vi "2025_day1.vi"() -> ()   [LabVIEW 2025]
uses:
  <userlib>/_OpenG.lib/string/string.llb/openg_string.lvlib
panel:
  out "Task 2":i32
  out "Task 1":i32
  in  "Switch":bool caption="Ex. Data  vs.  User Data"
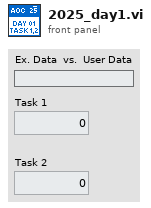
[diagram p1: front panel]
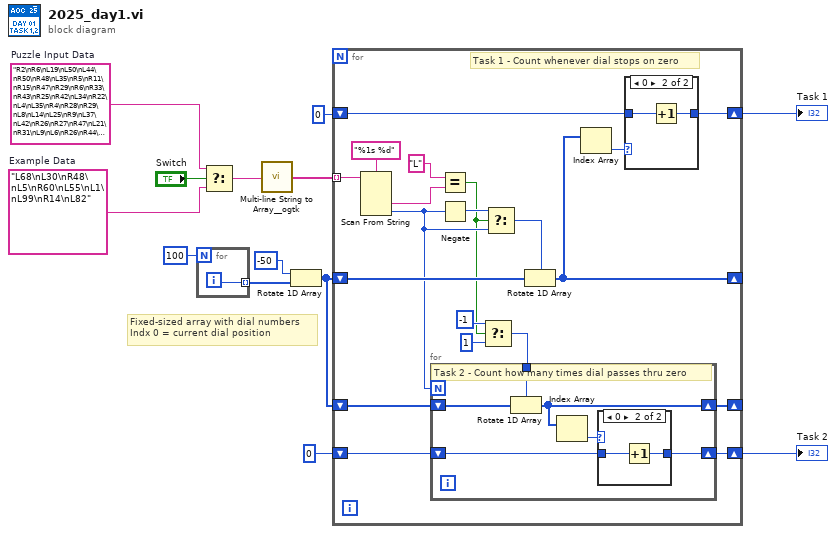
[diagram p0: block diagram]
diagram:
  w11 = "R2\nR6\nL19\nL50\nL44\nR50\nR48\nL35\nR5\nR11\nR15\nR47\nR29\nR6\nR33\nR43\nR25\nR42\nL34\nR22\nL4\nL35\nR4\nR28\nR29\nL8\nL14\nL25\nR9\nL37\nL42\nR26\nR27\nR47\nL21\nR31\nL9\nL6\nR26\nR44\nR2\nL38\nL14\nR21\nR49\nL47\nR23\nL25\nR20\nL13\nR12\nL46\nL66\nR12\nL41\nL92\nR19\nL89\nR30\nL39\nL30\nL24\nR13\nR75\nL92\nR58\nR68\nR32\nR12\nL33\nR49\nL28\nR41\nR24\nR76\nL62\nR14\nL93\nR25\nR75\nR68\nL19\nL49\nR13\nR71\nR16\nL4\nL40\nR31\nL75\nL90\nL40\nL82\nR63\nL99\nL56\nR17\nR40\nR94\nL59\nR12\nL3\nR91\nR66\nR34\nR525\nL325\nR53\nR168\nL212\nR291\nL16\nR81\nL65\nL37\nR76\nR25\nL64\nR10\nL310\nR28\nR42\nL70\nL984\nL59\nR159\nR54\nR30\nL39\nR19\nL880\nL824\nL64\nL22\nR10\nR20\nL17\nL103\nR3\nR82\nL85\nL30\nR35\nL605\nL75\nL44\nR19\nR88\nR12\nL35\nR4..."  # Puzzle Input Data
  w12 = "L68\nL30\nR48\nL5\nR60\nL55\nL1\nL99\nR14\nL82"  # Example Data
  # "Fixed-sized array with dial numbers\nIndx 0 = current dial position"
  n1 = for {
    N: 100 -> [_]
    tunnel: [w14] -> w7 mode=indexing
    i -> [w14]
  }
  n2 = Select(t=w11, s="Switch", f=w12) -> (s? t:f=w10:string)
  n3 = call <userlib>:"Multi-line String to Array__ogtk.vi"("string"=w10) -> ("lines"=w9:string[])
  n4 = Rotate 1D Array(1:w7, 2:-50 ("n")) -> (0:w3:i32[])
  n5 = for {
    tunnel: w9 -> [w34] mode=indexing
    shift-right: [w28] -> _
    shift-left: w3 -> [w24]
    shift-right: [w26] -> w4
    shift-left: 0 ("n") -> [w25]
    shift-right: [w22] -> _
    shift-left: w3 -> [w23]
    shift-right: [w16] -> w1
    shift-left: 0 ("n") -> [w15]
    # "Task 1 - Count whenever dial stops on zero"
    n6 = Scan From String(format string="%1s %d", input string=w34) -> (output 1=w31:string, output 2=w21:i32)  [unwired: 4 in, 3 out]
    n7 = Equal?(x="L", y=w31) -> (x = y?=w18:bool)
    n8 = Negate(x=w21) -> (-x=w32:i32)
    n9 = Select(t=-1, s=w18, f=1) -> (s? t:f=w17:i32)
    n10 = for {
      N: w21 -> [_]
      shift-right: [w35] -> w22
      shift-left: w23 -> [w40]
      tunnel: w17 -> [w39]
      shift-right: [w36] -> w16
      shift-left: w15 -> [w37]
      # "Task 2 - Count how many times dial passes thru zero"
      n11 = Rotate 1D Array(1:w40, 2:w39) -> (0:w35:i32[])
      n12 = Index Array(array=w35) -> (element=w38:i32)  [unwired: 1 in]
      n13 = case shown="0" w38 {
        tunnel: [w41 w42] -> w36
        tunnel: w37 -> [w41 w43]
        frame Default {
        }
        frame 0 {
          n14 = Increment(x=w43) -> (x+1=w42:i32)
        }
      }
    }
    n15 = Select(t=w32, s=w18, f=w21) -> (s? t:f=w29:i32)
    n16 = Rotate 1D Array(1:w24, 2:w29) -> (0:w28:i32[])
    n17 = Index Array(array=w28) -> (element=w27:i32)  [unwired: 1 in]
    n18 = case shown="0" w27 {
      tunnel: [w44 w45] -> w26
      tunnel: w25 -> [w44 w46]
      frame Default {
      }
      frame 0 {
        n19 = Increment(x=w46) -> (x+1=w45:i32)
      }
    }
  }
  "Task 1" <- w4
  "Task 2" <- w1
